vi "banner.vi"() -> ()   [LabVIEW 2017]
doc: "Illustrates setting the client banner and reading the server banner."
uses:
  libssh2/libssh2_session_handshake_tcp.vi
  libssh2/libssh2_init_default.vi
  libssh2/libssh2_session_init_ex.vi
  <vilib>/Utility/tcp.llb/TCP Get Raw Net Object.vi
  libssh2/libssh2_session_handshake_socket.vi
  libssh2/libssh2.lvlib
panel:
  in  "client banner":string="SSH-2.0-libssh2_1.11.0"
  out "server banner":string
  out "error out":errorcluster
  in  "hostname":string="localhost"
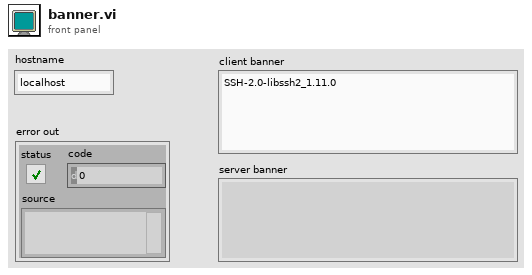
[diagram p1: front panel]
types:
  T1 = typedef "libssh2.lvlib/Session Refnum.ctl" = refnum<k1>
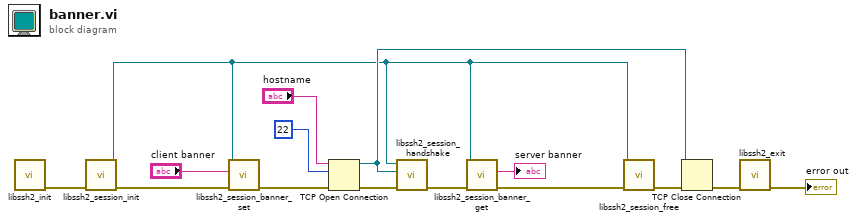
[diagram p0: block diagram]
diagram:
  n1 = call-poly "libssh2_init.vi"() -> ("error out"=w15:errorcluster)  [unwired: 11 in]
  n2 = call "libssh2_session_init.vi"("error in (no error)"=w15) -> ("error out"=w3:errorcluster, "session"=w5:T1)  [unwired: 9 in]
  n3 = call "libssh2_session_banner_set.vi"("error in (no error)"=w3, "banner"="client banner", "session"=w5) -> ("error out"=w2:errorcluster)  [unwired: 8 in]
  n4 = TCP Open Connection(address="hostname", remote port or service name=u16 22, error in (no error)=w2) -> (connection ID=w9:refnum<k5>, error out=w10:errorcluster)  [unwired: 2 in]
  n5 = call-poly "libssh2_session_handshake.vi"("error in (no error)"=w10, "tcp connection"=w9, "session"=w5) -> ("error out"=w1:errorcluster)  [unwired: 8 in]
  n6 = call "libssh2_session_banner_get.vi"("error in (no error)"=w1, "session"=w5) -> ("error out"=w7:errorcluster, "banner"=→"server banner":string)  [unwired: 8 in]
  n7 = call "libssh2_session_free.vi"("error in (no error)"=w7, "session"=w5) -> ("error out"=w14:errorcluster)  [unwired: 9 in]
  n8 = TCP Close Connection(connection ID=w9, error in (no error)=w14) -> (error out=w11:errorcluster)  [unwired: 1 in, 1 out]
  n9 = call "libssh2_exit.vi"("error in (no error)"=w11) -> ("error out"=→"error out":errorcluster)  [unwired: 10 in]
